vi "Configure Generation.vi"(8 "error in":errorcluster, 11 "DO DAQmx Fixed Freq PWM CFG in":refnum<class "DO DAQmx Fixed Freq PWM CFG.lvclass">) -> (0 "error out":errorcluster, 3 "DO DAQmx Fixed Freq PWM CFG out":refnum<class "DO DAQmx Fixed Freq PWM CFG.lvclass">)   [LabVIEW 2023, in "DO DAQmx Fixed Freq PWM CFG.lvclass"]
uses:
  DO DAQmx Fixed Freq PWM CFG.lvclass
  DO DAQmx Fixed Freq PWM CFG.lvclass/DO DAQmx Fixed Freq PWM CFG.ctl
  DAQmx/DAQmx Base CFG/DAQmx Base CFG.lvclass
  <resource>/objmgr/daqmx.rc
  Configuration/Configuration JSON/Configuration JSON Base/CFG JSON.lvclass
  <vilib>/ErrorRing/Error Ring.xnode
  <vilib>/Utility/error.llb/Error Cluster From Error Code.vi
  <vilib>/DAQmx/write.llb/DAQmx Write (Digital 1D Wfm NChan NSamp).vi
  936b0159-b9c4-4cd4-83f0-0b0335a34480.vi
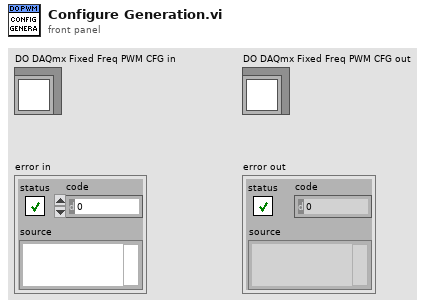
[diagram p1: front panel]
types:
  T1 = cluster{"Channel":string, "Digital Waveform":digitalwaveform}[]
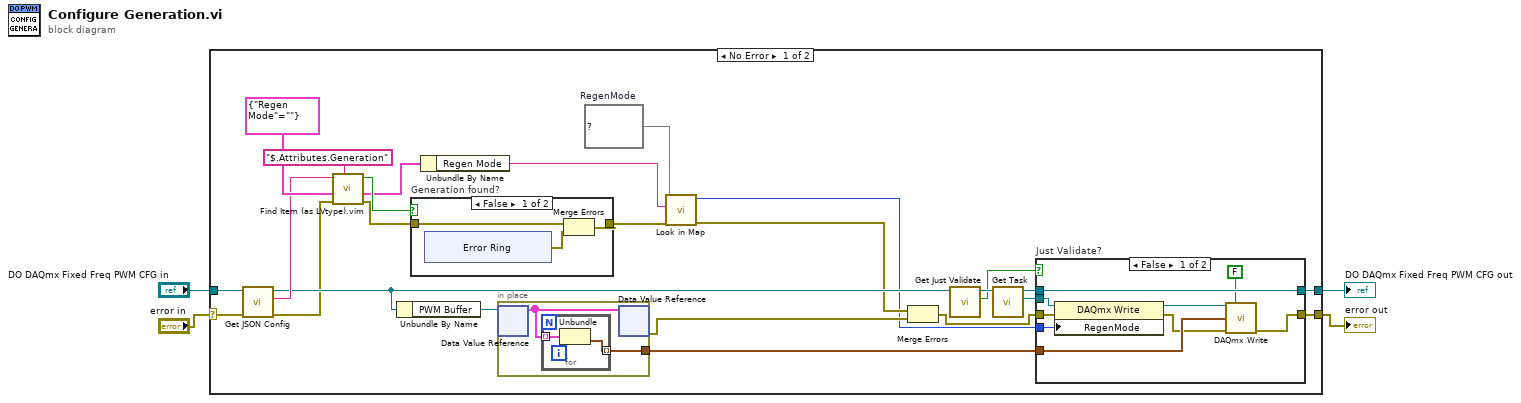
[diagram p0: block diagram]
diagram:
  n1 = case shown="No Error" "error in" {
    selector: "error in" -> [w10 w54]
    tunnel: [w16 w54] -> w3
    tunnel: [w17 w53] -> w1
    tunnel: "DO DAQmx Fixed Freq PWM CFG in" -> [w27 w53]
    frame No Error {
      w9 = map{string, i32} {"Allow Regeneration"=10097, "Do Not Allow Regeneration"=10158}  # RegenMode
      n2 = call "Get JSON Config.vi"("CFG Base in"=w27) -> ("<JSON>Config>"=w21:string, "CFG Base out"=w15:refnum<class "DO DAQmx Fixed Freq PWM CFG.lvclass">)  [unwired: 9 in]
      n3 = call "Find Item (as LVtype).vim"("$Path or Item Name"="$.Attributes.Generation", "error in (no error)"=w10, "Data Type and Default Value"=cluster{"Regen Mode":string} {"Regen Mode"=""}, "JSON"=w21) -> ("error out"=w26:errorcluster, "Data"=w22:cluster{"Regen Mode":string}, "Found"=w25:bool)  [unwired: 4 in, 1 out]
      n4 = Unbundle By Name(w15) -> ("PWM Buffer"=w14:refnum<data-value>)
      n5 = case "Generation found?" shown="False" w25 {
        tunnel: w26 -> [w46 w52]
        tunnel: [w44 w52] -> w7
        frame False {
          n6 = xnode "Error Ring"() -> ("error out"=w45:errorcluster)
          n7 = Merge Errors(w46, w45) -> (w44:errorcluster)
        }
        frame True {
        }
      }
      n8 = Unbundle By Name(w22) -> ("Regen Mode"=w8:string)
      n9 = in-place {
        in-place-border: [w29] -> w13
        n10 = in-place-dvr #1(w14) -> (w30:T1)  [unwired: 1 out]
        n11 = for {
          tunnel: w30 -> [w32] mode=indexing
          tunnel: [w31] -> w29 mode=indexing
          n12 = Unbundle(w32) -> ("Digital Waveform"=w31:digitalwaveform)  [unwired: 1 out]
        }
        n13 = in-place-dvr #1(w30) -> (w12:errorcluster)  [unwired: 1 out]
      }
      n14 = call "Look in Map.vi"("error in"=w7, "Key"=w8, "Map"=w9) -> ("error out"=w6:errorcluster, "Value"=w5:i32)  [unwired: 7 in]
      n15 = Merge Errors(w6, w12) -> (w11:errorcluster)
      n16 = call "Get Just Validate.vi"("CFG JSON Base in"=w15) -> ("Just Validate"=w19:bool, "CFG JSON Base out"=w20:refnum<class "DO DAQmx Fixed Freq PWM CFG.lvclass">)  [unwired: 9 in]
      n17 = call "Get Task.vi"("DAQmx Base CFG in"=w20) -> ("Task"=w28:refnum<k21>, "DAQmx Base CFG out"=w18:refnum<class "DO DAQmx Fixed Freq PWM CFG.lvclass">)  [unwired: 9 in]
      n18 = case "Just Validate?" shown="False" w19 {
        tunnel: w11 -> [w41 w42]
        tunnel: w28 -> [w40 _]
        tunnel: w5 -> [w39 _]
        tunnel: w18 -> [w34 w43]
        tunnel: [w34 w43] -> w17
        tunnel: [w35 w42] -> w16
        tunnel: w13 -> [w37 _]
        frame False {
          n19 = property class="DAQmx Write"(reference=w40, error in=w41, "RegenMode"=w39) -> (reference out=w38:refnum<k21>, error out=w36:errorcluster)
          n20 = call-poly <vilib>:"DAQmx Write.vi"("task/channels in"=w38, "auto start"=FALSE, "data"=w37, "error in"=w36) -> ("error out"=w35:errorcluster)  [unwired: 9 in, 2 out]
        }
        frame True {
        }
      }
    }
    frame Error {
    }
  }
  "error out" <- w3
  "DO DAQmx Fixed Freq PWM CFG out" <- w1
